vi "Write Executor Number.vi"(8 "error in (no error)":errorcluster, 10 "Executor Number":i32, 11 "Job in":refnum<class "Job.lvclass">) -> (0 "error out":errorcluster, 3 "Job out":refnum<class "Job.lvclass">)   [LabVIEW 2014, in "Job.lvclass"]
uses:
  Job.lvclass
  Job.lvclass/Job.ctl
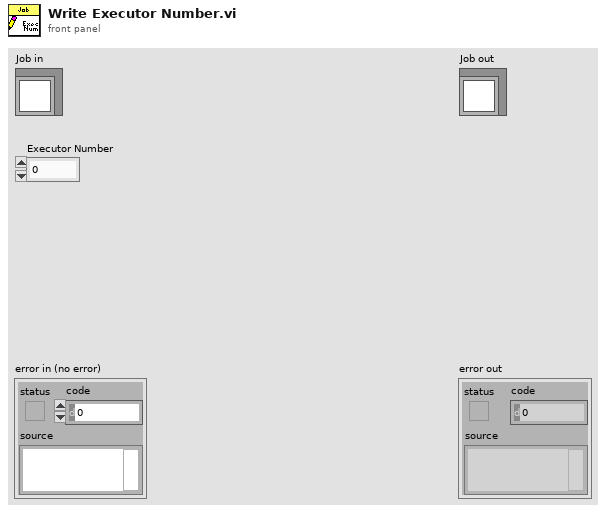
[diagram p1: front panel]
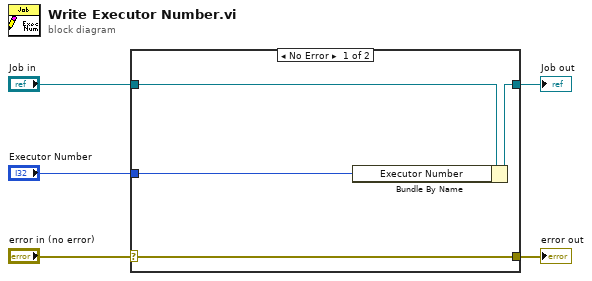
[diagram p0: block diagram]
diagram:
  n1 = case shown="No Error" "error in (no error)" {
    selector: "error in (no error)" -> [w9 w10]
    tunnel: [w9 w10] -> w4
    tunnel: [w7 w11] -> w2
    tunnel: "Job in" -> [w8 w11]
    tunnel: "Executor Number" -> [w6 _]
    frame No Error {
      n2 = Bundle By Name(cluster=w8, "Executor Number"=w6) -> (w7:refnum<class "Job.lvclass">)
    }
    frame Error {
    }
  }
  "error out" <- w4
  "Job out" <- w2
